vi "Execute_State.vi"(8 "error in":errorcluster, 10 "State_Info":T1, 11 "Parameters to process":T5) -> (0 "error out":errorcluster, 2 "State_Info_Out":T1)   [LabVIEW 2017, in "ExampleSequencer runtime.lvclass"]
uses:
  ExampleSequencer runtime.lvclass
  parameter user data.ctl
  State.ctl
  Utilities/StateMachine.ctl
  <vilib>/NI/STM/TCP/TCP Connection Info.ctl
  <vilib>/NI/STM/SubVIs/MetaDataElement.ctl
  <vilib>/NI/STM/TCP/TCP Write Options.ctl
  Utilities/Controlword_Commands.ctl
  Utilities/Controlword_ReadMode.ctl
  <vilib>/NI/STM/TCP/Write Meta Data (TCP Ref).vi
  <vilib>/NI/STM/TCP/Write Meta Data (TCP Clst).vi
  <vilib>/NI/STM/TCP/Read Message (TCP).vi
  <vilib>/NI/STM/TCP/Write Message (TCP).vi
  <vilib>/NI/STM/NI STM.lvlib
  Utilities/WordManipulationLibrary.lvlib
  Utilities/Bit Manipulation.lvlib
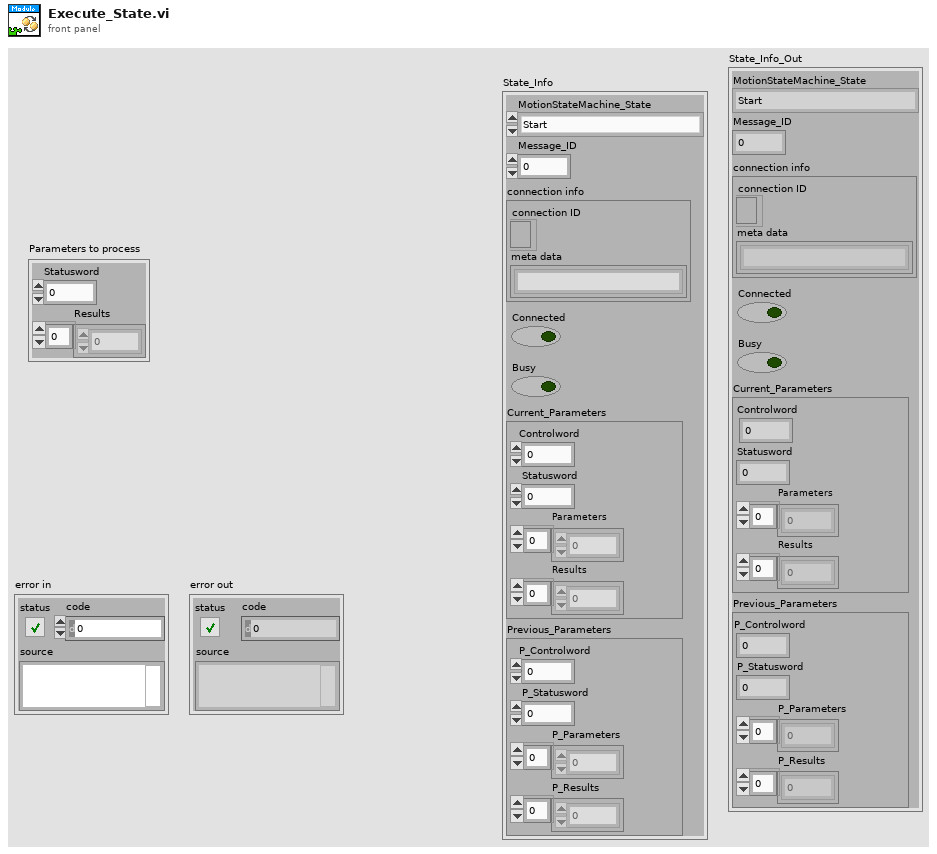
[diagram p1: front panel]
types:
  T1 = typedef "State.ctl" = cluster{"MotionStateMachine_State":T2, "Message_ID":u32, "connection info":T3, "Connected":bool, "Busy":bool, "Current_Parameters":cluster{"Controlword":u16, "Statusword":u16, "Parameters":dbl[], "Results":dbl[]}, "Previous_Parameters":cluster{"P_Controlword":u16, "P_Statusword":u16, "P_Parameters":dbl[], "P_Results":dbl[]}}
  T2 = typedef "WordManipulationLibrary.lvlib/StateMachine.ctl" = enum16{"Start", "Not Ready to Switch On", "Switch On Disabled", "Ready to Switch On", "Switched On", "Operation enable", "Quick Stop Active", "Fault Reaction Active", "Fault"}
  T3 = typedef "NI STM.lvlib/TCP Connection Info.ctl" = cluster{"connection ID":refnum<k5>, "meta data":T4[]}
  T4 = typedef "NI STM.lvlib/MetaDataElement.ctl" = string
  T5 = typedef "ExampleSequencer runtime.lvclass/parameter user data.ctl" = cluster{"Statusword":u16, "Results":dbl[]}
  T6 = typedef "NI STM.lvlib/TCP Write Options.ctl" = cluster{"ignore timeout error":bool, "timeout ms (1000)":i32}
  T7 = typedef "WordManipulationLibrary.lvlib/Controlword_Commands.ctl" = enum16{"Shutdown", "Switch On", "Disable Voltage", "Quick Stop", "Disable Op", "Enable Op", "Fault Reset", "Error"}
  T8 = typedef "WordManipulationLibrary.lvlib/Controlword_ReadMode.ctl" = enum16{"Fast Read", "Full Read", "Full Read With Fault Check"}
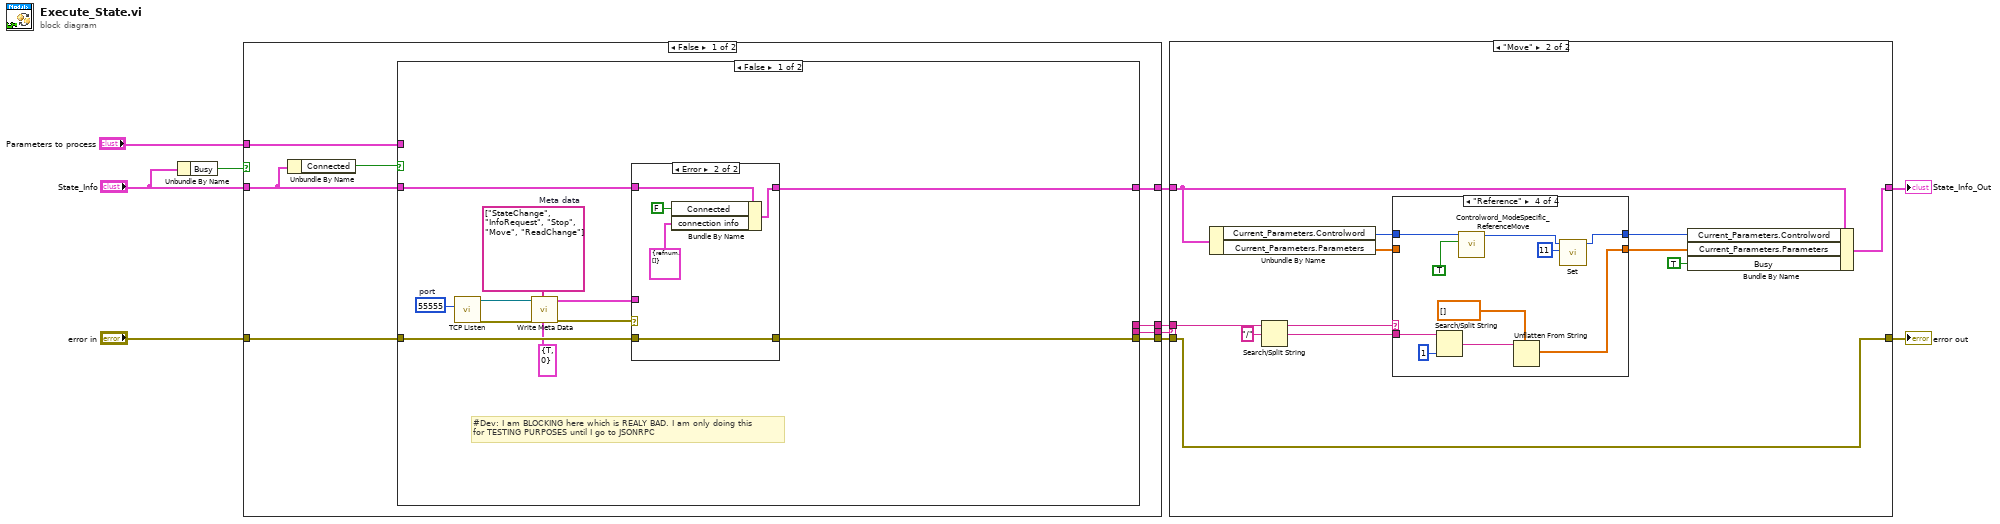
[diagram p0: block diagram]
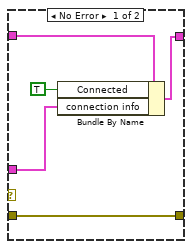
[diagram p2: hidden frame]
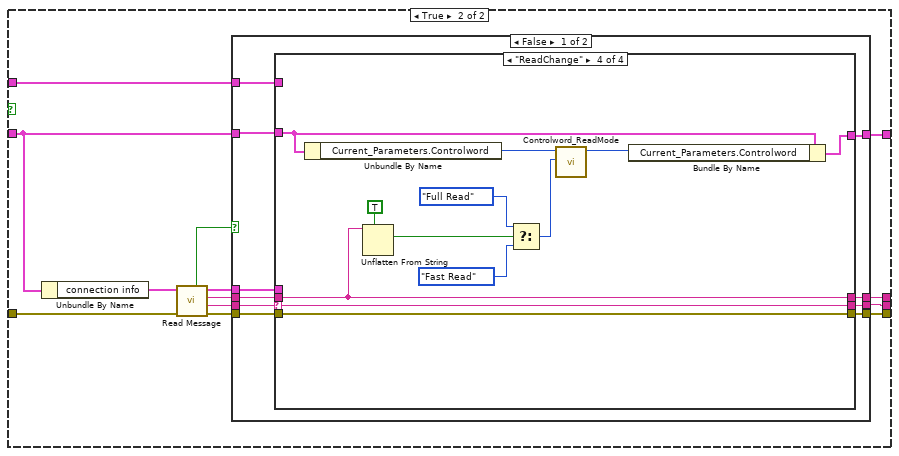
[diagram p3: hidden frame]
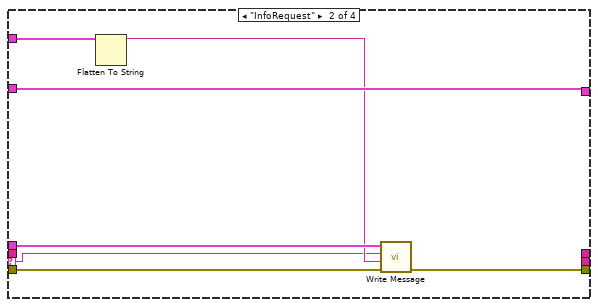
[diagram p5: hidden frame]
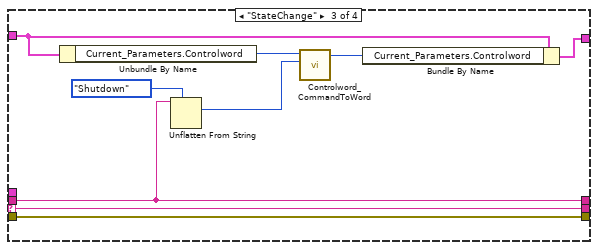
[diagram p6: hidden frame]
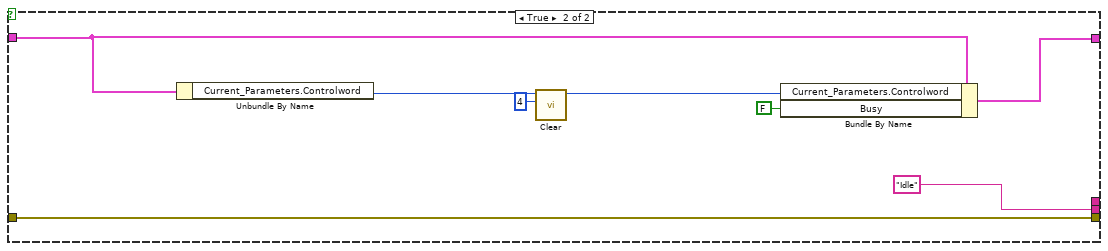
[diagram p8: hidden frame]
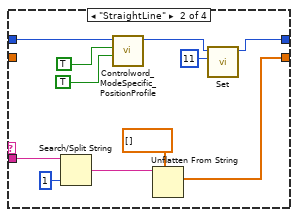
[diagram p11: hidden frame]
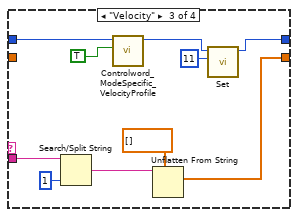
[diagram p12: hidden frame]
diagram:
  n1 = Unbundle By Name("State_Info") -> ("Busy"=w3:bool)
  n2 = case shown="False" w3 {
    tunnel: "error in" -> [w17 w105]
    tunnel: "State_Info" -> [w16 w103]
    tunnel: [w15 "Idle"] -> w9
    tunnel: [w14 w102] -> w8
    tunnel: [w13 w105] -> w7
    tunnel: [w12 _] -> w2
    tunnel: "Parameters to process" -> [w11 _]
    frame False {
      n3 = Unbundle By Name(w16) -> ("Connected"=w18:bool)
      n4 = case shown="False" w18 {
        tunnel: w17 -> [w23 w52]
        tunnel: w16 -> [w25 w45]
        tunnel: [w22 w49] -> w13
        tunnel: [w21 w44] -> w14
        tunnel: [_ w43] -> w15
        tunnel: [_ w42] -> w12
        tunnel: w11 -> [_ w40]
        frame False {
          w29 = T4[] ["StateChange", "InfoRequest", "Stop", "Move", "ReadChange"]  # Meta data
          w27 = u16 55555  # port
          # "#Dev: I am BLOCKING here which is REALY BAD. I am only doing this \nfor TESTING PURPOSES until I go to JSONRPC"
          n5 = call <vilib>:"TCP Listen.vi"("port"=w27) -> ("error out"=w28:errorcluster, "connection ID"=w19:refnum<k5>)  [unwired: 3 in, 6 out]
          n6 = call-poly <vilib>:"Write Meta Data.vi"("options"=T6 {"ignore timeout error"=TRUE, "timeout ms (1000)"=0}, "meta data"=w29, "error in"=w28, "connection ID"=w19) -> ("error out"=w26:errorcluster, "connection info out"=w24:T3)  [unwired: 1 in, 5 out]
          n7 = case shown="Error" w26 {
            tunnel: w25 -> [w34 w37]
            tunnel: w24 -> [w32 _]
            tunnel: w23 -> [w31 w35]
            tunnel: [w31 w35] -> w22
            tunnel: [w30 w36] -> w21
            frame No Error {
              n8 = Bundle By Name(cluster=w34, "Connected"=TRUE, "connection info"=w32) -> (w30:T1)
            }
            frame Error {
              n9 = Bundle By Name(cluster=w37, "Connected"=FALSE, "connection info"=T3 {"connection ID"=refnum, "meta data"=[]}) -> (w36:T1)
            }
          }
        }
        frame True {
          n10 = Unbundle By Name(w45) -> ("connection info"=w51:T3)
          n11 = call-poly <vilib>:"Read Message.vi"("error in"=w52, "connection info in"=w51) -> ("error out"=w48:errorcluster, "name"=w47:T4, "data string"=w46:string, "connection info out"=w41:T3, "timed out?"=w50:bool)  [unwired: 3 in, 2 out]
          n12 = case shown="False" w50 {
            tunnel: [w60 w97] -> w49
            tunnel: w48 -> [w62 w97]
            tunnel: w47 -> [w61 _]
            tunnel: w46 -> [w58 w95]
            tunnel: w45 -> [w59 w96]
            tunnel: [w57 w96] -> w44
            tunnel: [w56 _] -> w43
            tunnel: [w55 w95] -> w42
            tunnel: w41 -> [w54 _]
            tunnel: w40 -> [w53 _]
            frame False {
              n13 = case shown="\"ReadChange\"" w61 {
                selector: w61 -> [w64 w67 w75 w91]
                tunnel: w62 -> [w66 w73 w77 w92]
                tunnel: [w66 w72 w77 w92] -> w60
                tunnel: w59 -> [w65 w70 w79 w93]
                tunnel: w58 -> [w63 _ w74 w90]
                tunnel: [w65 w70 w80 w94] -> w57
                tunnel: [w64 _ w75 w91] -> w56
                tunnel: [w63 _ w74 w90] -> w55
                tunnel: w54 -> [_ w71 _ _]
                tunnel: w53 -> [_ w69 _ _]
                frame "False", Default {
                }
                frame "InfoRequest" {
                  n14 = Flatten To String(anything=w69) -> (data string=w68:string)  [unwired: 3 in, 2 out]
                  n15 = call-poly <vilib>:"Write Message.vi"("error in"=w73, "data"=w68, "name"=w67, "connection info in"=w71) -> ("error out"=w72:errorcluster)  [unwired: 6 in, 1 out]
                }
                frame "StateChange" {
                  n16 = Unbundle By Name(w79) -> ("Current_Parameters.Controlword"=w81:u16)
                  n17 = Unflatten From String(type=Controlword_Commands."Shutdown" ("Device Control Command"), binary string=w74) -> (value=w76:T7)  [unwired: 3 in, 2 out]
                  n18 = call "Controlword_CommandToWord.vi"("Device Control Command"=w76, "ControlWord In"=w81) -> ("ControlWord Out"=w78:u16)  [unwired: 9 in]
                  n19 = Bundle By Name(cluster=w79, "Current_Parameters.Controlword"=w78) -> (w80:T1)
                }
                frame "ReadChange" {
                  n20 = Unbundle By Name(w93) -> ("Current_Parameters.Controlword"=w88:u16)
                  n21 = Unflatten From String(type=TRUE, binary string=w90) -> (value=w83:bool)  [unwired: 3 in, 2 out]
                  n22 = Select(t=Controlword_ReadMode."Full Read" ("Read mode"), s=w83, f=Controlword_ReadMode."Fast Read" ("Read mode")) -> (s? t:f=w84:T8)
                  n23 = call "Controlword_ReadMode.vi"("Read mode"=w84, "ControlWord In"=w88) -> ("ControlWord Out"=w87:u16)  [unwired: 9 in]
                  n24 = Bundle By Name(cluster=w93, "Current_Parameters.Controlword"=w87) -> (w94:T1)
                }
              }
            }
            frame True {
            }
          }
        }
      }
    }
    frame True {
      n25 = Unbundle By Name(w103) -> ("Current_Parameters.Controlword"=w101:u16)
      n26 = call "Clear.vi"("Bit to clear"=u8 4, "Data_In"=w101) -> ("Data_Out"=w100:u16)  [unwired: 9 in]
      n27 = Bundle By Name(cluster=w103, "Current_Parameters.Controlword"=w100, "Busy"=FALSE) -> (w102:T1)
    }
  }
  n28 = case shown="\"Move\"" w9 {
    tunnel: w8 -> [w106 w118]
    tunnel: w7 -> [w107 w108]
    tunnel: [w107 w108] -> w6
    tunnel: [w106 w119] -> w5
    tunnel: w2 -> [_ w117]
    frame "Idle", Default {
    }
    frame "Move" {
      n29 = Unbundle By Name(w118) -> ("Current_Parameters.Controlword"=w112:u16, "Current_Parameters.Parameters"=w109:dbl[])
      n30 = Search/Split String(string=w117, search string/char (-)="/") -> (substring before match=w115:string, match + rest of string=w114:string)  [unwired: 1 in, 1 out]
      n31 = case shown="\"Reference\"" w115 {
        tunnel: w114 -> [_ w132 w142 w152]
        tunnel: [w120 w128 w138 w147] -> w113
        tunnel: w112 -> [w121 w127 w135 w145]
        tunnel: [w121 w123 w137 w149] -> w111
        tunnel: w109 -> [w120 _ _ _]
        frame "False", Default {
        }
        frame "StraightLine" {
          n32 = Search/Split String(string=w132, offset (0)=1) -> (match + rest of string=w130:string)  [unwired: 1 in, 2 out]
          n33 = call "Controlword_ModeSpecific_PositionProfile.vi"("Change Immediately? (If False, will Blend)"=TRUE, "New Setpoint?"=TRUE, "ControlWord In"=w127) -> ("ControlWord Out"=w124:u16)  [unwired: 8 in]
          n34 = Unflatten From String(type=dbl[] [], binary string=w130) -> (value=w128:dbl[])  [unwired: 3 in, 2 out]
          n35 = call "Set.vi"("Bit to set"=u8 11, "Data_In"=w124) -> ("Data_Out"=w123:u16)  [unwired: 9 in]
        }
        frame "Velocity" {
          n36 = Search/Split String(string=w142, offset (0)=1) -> (match + rest of string=w140:string)  [unwired: 1 in, 2 out]
          n37 = call "Controlword_ModeSpecific_VelocityProfile.vi"("New Setpoint?"=TRUE, "ControlWord In"=w135) -> ("ControlWord Out"=w134:u16)  [unwired: 9 in]
          n38 = Unflatten From String(type=dbl[] [], binary string=w140) -> (value=w138:dbl[])  [unwired: 3 in, 2 out]
          n39 = call "Set.vi"("Bit to set"=u8 11, "Data_In"=w134) -> ("Data_Out"=w137:u16)  [unwired: 9 in]
        }
        frame "Reference" {
          n40 = Search/Split String(string=w152, offset (0)=1) -> (match + rest of string=w150:string)  [unwired: 1 in, 2 out]
          n41 = call "Controlword_ModeSpecific_ReferenceMove.vi"("Operation Start"=TRUE, "ControlWord In"=w145) -> ("ControlWord Out"=w144:u16)  [unwired: 9 in]
          n42 = Unflatten From String(type=dbl[] [], binary string=w150) -> (value=w147:dbl[])  [unwired: 3 in, 2 out]
          n43 = call "Set.vi"("Bit to set"=u8 11, "Data_In"=w144) -> ("Data_Out"=w149:u16)  [unwired: 9 in]
        }
      }
      n44 = Bundle By Name(cluster=w118, "Current_Parameters.Controlword"=w111, "Current_Parameters.Parameters"=w113, "Busy"=TRUE) -> (w119:T1)
    }
  }
  "error out" <- w6
  "State_Info_Out" <- w5
